vi "Render Glyph.vi"(8 "error in (no error)":errorcluster, 9 "Colors":T1, 10 "glyph ref in":i64, 11 "Freetype Drawer in":refnum<class "Freetype Drawer.lvclass">) -> (0 "error out":errorcluster, 1 "image data":T2, 2 "glyph ref out":i64, 3 "Freetype Drawer out":refnum<class "Freetype Drawer.lvclass">)   [LabVIEW 2023, in "Freetype Drawer.lvlib" / "Freetype Drawer.lvclass"]
uses:
  Freetype Drawer.lvclass
  <vilib>/picture/picture.llb/imagedata.ctl
  Freetype Drawer.lvclass/Freetype Drawer.ctl
  Freetype Drawer.lvlib
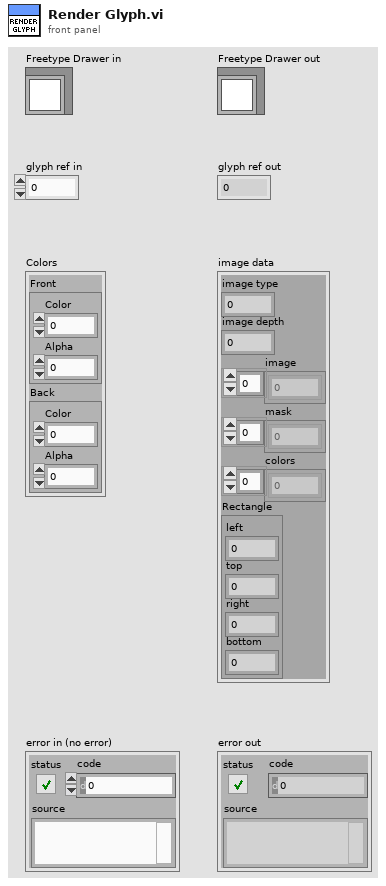
[diagram p1: front panel]
types:
  T1 = cluster{"Front":cluster{"Color":u32, "Alpha":u8}, "Back":cluster{"Color":u32, "Alpha":u8}}
  T2 = typedef "imagedata.ctl" = cluster{"image type":i32, "image depth":i32, "image":u8[], "mask":u8[], "colors":u32[], "Rectangle":cluster{"left":i16, "top":i16, "right":i16, "bottom":i16}}
  T3 = cluster{"Width":i16, "Style":enum32{"Solid", "Dash", "Dot", "DashDot", "DashDotDot"}}
  T4 = cluster{"left":i16, "top":i16, "right":i16, "bottom":i16}
  T5 = typedef "Freetype Drawer.lvlib/Bitmap Glyph.ctl" = cluster{"root":T6, "left":i32, "top":i32, "bitmap":T7}
  T6 = typedef "Freetype Drawer.lvlib/Glyph Rec.ctl" = cluster{"library ref":i64, "class ref":i64, "format":i32, "advance":cluster{"x":i32, "y":i32}}
  T7 = typedef "Freetype Drawer.lvlib/FT Bitmap.ctl" = cluster{"rows":u32, "width":u32, "pitch":i32, "buffer ref":i64, "num grays":i16, "pixel_mode":u8, "palette mode":u8, "palette":i64}
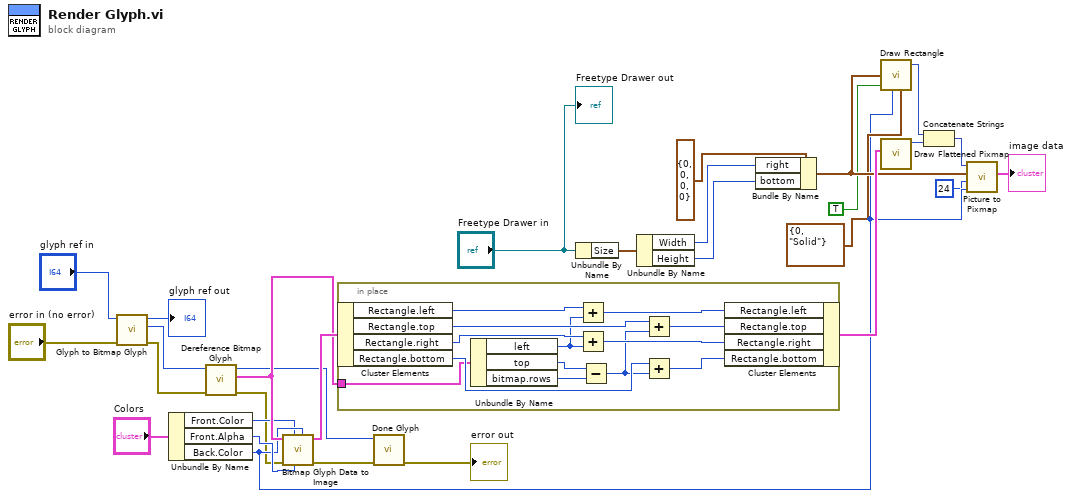
[diagram p0: block diagram]
diagram:
  n1 = call "Glyph to Bitmap Glyph.vi"("error in (no error)"="error in (no error)", "glyph ref in"="glyph ref in") -> ("error out"=w23:errorcluster, "bitmap glyph ref out"=w24:i64, "glyph ref out"=→"glyph ref out":i64)  [unwired: 7 in]
  n2 = Unbundle By Name("Colors") -> ("Front.Color"=w8:u32, "Front.Alpha"=w28:u8, "Back.Color"=w17:u32)
  n3 = call "Dereference Bitmap Glyph.vi"("error in (no error)"=w23, "glyph ref in"=w24) -> ("error out"=w5:errorcluster, "Bitmap Glyph Rec"=w22:T5, "glyph ref out"=w4:i64)  [unwired: 7 in]
  n4 = call "Bitmap Glyph Data to Image.vi"("Back"=w17, "Alpha"=w28, "Front"=w8, "error in (no error)"=w5, "Bitmap Glyph Rec"=w22) -> ("error out"=w6:errorcluster, "image data"=w26:T2)  [unwired: 5 in]
  n5 = in-place {
    in-place-border: w22 -> [w30]
    n6 = in-place-cluster #1(w26) -> ("Rectangle.left"=w42:i16, "Rectangle.top"=w41:i16, "Rectangle.right"=w40:i16, "Rectangle.bottom"=w39:i16)
    n7 = Unbundle By Name(w30) -> ("left"=w34:i32, "top"=w33:i32, "bitmap.rows"=w31:u32)
    n8 = Add(x=w42, y=w34) -> (x+y=w38:i32)
    n9 = Add(x=w40, y=w34) -> (x+y=w36:i32)
    n10 = Subtract(x=w33, y=w31) -> (x-y=w32:u32)
    n11 = Add(x=w41, y=w32) -> (x+y=w37:u32)
    n12 = Add(x=w39, y=w32) -> (x+y=w35:u32)
    n13 = in-place-cluster #1("Rectangle.left"=w38, "Rectangle.top"=w37, "Rectangle.right"=w36, "Rectangle.bottom"=w35) -> (w21:T2)
  }
  n14 = call "Done Glyph.vi"("error in (no error)"=w6, "glyph ref in"=w4) -> ("error out"=→"error out":errorcluster)  [unwired: 9 in]
  n15 = Unbundle By Name("Freetype Drawer in") -> ("Size"=w29:cluster{"Width":u16, "Height":u16})
  n16 = Unbundle By Name(w29) -> ("Width"=w10:u16, "Height"=w11:u16)
  n17 = Bundle By Name(cluster=T4 {"left"=0, "top"=0, "right"=0, "bottom"=0} ("rect"), "right"=w10, "bottom"=w11) -> (w20:T4)
  n18 = call <vilib>:"Draw Rectangle.vi"("rect"=w20, "fill?(F)"=TRUE, "color(black)"=w17, "pen"=T3 {"Width"=0, "Style"=enum."Solid"}) -> ("new picture"=w16:picture)  [unwired: 5 in]
  n19 = call <vilib>:"Draw Flattened Pixmap.vi"("image data"=w21) -> ("new picture"=w12:picture)  [unwired: 8 in]
  n20 = Concatenate Strings(w16, w12) -> (w15:picture)
  n21 = call <vilib>:"Picture to Pixmap.vi"("Background Color"=w17, "depth"=24, "rect"=w20, "picture"=w15) -> ("image data"=→"image data":T2)  [unwired: 6 in, 1 out]
  "Freetype Drawer out" <- "Freetype Drawer in"
